vi "Teleop.vi"(10 "Match Info":T1={"Autonomous Elapsed Seconds"=0.0, "TeleOp Elapsed Seconds"=0.0, "Disabled Elapsed Seconds"=0.0, "Visited Autonomous"=FALSE, "Visited TeleOp"=FALSE, "Visited Disabled"=FALSE, "Autonomous Settings"={"Autonomous Style"=enum."Independent", "VI Refnum"=refnum}}, 11 "Call Context":T2) -> ()   [LabVIEW 2013]
doc: "This VI is called for each TeleOp packet received from the DS where the robot is not disabled. It is often used to read from the joysticks and update I/O or to update setpoints for timed control loops. It should complete and return within 20 milliseconds or it may miss DS packets."
uses:
  <vilib>/Rock Robotics/WPI/DriverStation/WPI_DriverStationDerivedRobotMode.ctl
  <vilib>/Rock Robotics/WPI/DriverStation/WPI_DriverStationMatch Info.ctl
  <vilib>/Rock Robotics/WPI/Joystick/WPI_JoystickAxis.ctl
  Robot Global Data.vi
  <vilib>/Rock Robotics/WPI/RobotDrive/WPI_RobotDriveMecanumDrive_Cartesian.vi
  <vilib>/Rock Robotics/WPI/Joystick/WPI_JoystickGetSetRefNum.vi
  <vilib>/Rock Robotics/WPI/RobotDrive/WPI_RobotDriveGetSetRefNum.vi
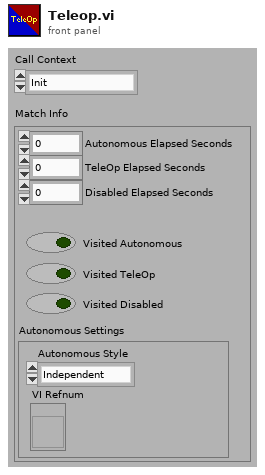
[diagram p1: front panel]
types:
  T1 = typedef "WPI_DriverStationMatch Info.ctl" = cluster{"Autonomous Elapsed Seconds":dbl, "TeleOp Elapsed Seconds":dbl, "Disabled Elapsed Seconds":dbl, "Visited Autonomous":bool, "Visited TeleOp":bool, "Visited Disabled":bool, "Autonomous Settings":cluster{"Autonomous Style":enum16{"Iterative", "Independent"}, "VI Refnum":refnum<vi>}}
  T2 = typedef "WPI_DriverStationDerivedRobotMode.ctl" = enum16{"Init", "Execute", "Stop"}
  T3 = typedef "WPI_JoystickAxis.ctl" = enum16{"Axis 1", "Axis 2", "Axis 3", "Axis 4", "Axis 5", "Axis 6"}
  T4 = typedef "WPI_JoystickDevRef.ctl" = cluster{"Device":T5}
  T5 = typedef "WPI_JoystickDeviceEnum.ctl" = enum16{"USB 1", "USB 2", "USB 3", "USB 4", "Kinect 1", "Kinect 2"}
  T6 = cluster{"axis 1 (x)":dbl, "axis 2 (y)":dbl, "axis 3 (throttle)":dbl, "axis 4":dbl, "axis 5":dbl, "axis 6":dbl}
  T7 = typedef "WPI_AnalogChannelDevRef.ctl" = cluster{"DevStatus":errorcluster, "Analog Module":T8, "Analog Channel":T9}
  T8 = typedef "FPGA_TypedefAnalogModule.ctl" = enum16{"Analog Module 1", "Analog Module 2"}
  T9 = typedef "FPGA_AIChannel.ctl" = enum8{"AI 1", "AI 2", "AI 3", "AI 4", "AI 5", "AI 6", "AI 7", "AI 8", "Invalid"}
  T10 = typedef "WPI_MotorControlDeviceRef.ctl" = cluster{"DeviceStatus":errorcluster, "Type":enum16{"PWM", "CAN"}, "PWM":cluster{"Digital Module":T11, "PWM Channel":T12, "DeadBand":T13}, "CAN":cluster{"Device Number":u8, "Control Mode":T14, "Semaphore":T15, "Max Vout":dbl}, "Invert":bool, "TransformRef":T16, "InvTransformRef":T16}
  T11 = typedef "FPGA_TypedefDigitalModule.ctl" = enum16{"Digital Module 1", "Digital Module 2"}
  T12 = typedef "FPGA_DIOPWMChannel.ctl" = enum8{"PWM 1", "PWM 2", "PWM 3", "PWM 4", "PWM 5", "PWM 6", "PWM 7", "PWM 8", "PWM 9", "PWM 10", "Invalid"}
  T13 = typedef "WPI_PWMDeadband.ctl" = cluster{"Name":string, "maxPositivePwm":i32, "minPositivePwm":i32, "centerPwm":i32, "maxNegativePwm":i32, "minNegativePwm":i32, "angularRange":u16}
  T14 = typedef "WPI_CANJaguar_ControlMode.ctl" = enum8{"Percent VBus", "Current", "Speed", "Position", "Voltage"}
  T15 = typedef "Semaphore RefNum" = refnum<k1>
  T16 = typedef "WPI_PWMTransform_ConPane.ctl" = refnum<vi>
  T17 = typedef "WPI_RobotDriveDevRef.ctl" = cluster{"DevStatus":errorcluster, "Motors[]":T10[], "Square Inputs":bool, "Max Output":dbl, "Isochronous":bool}
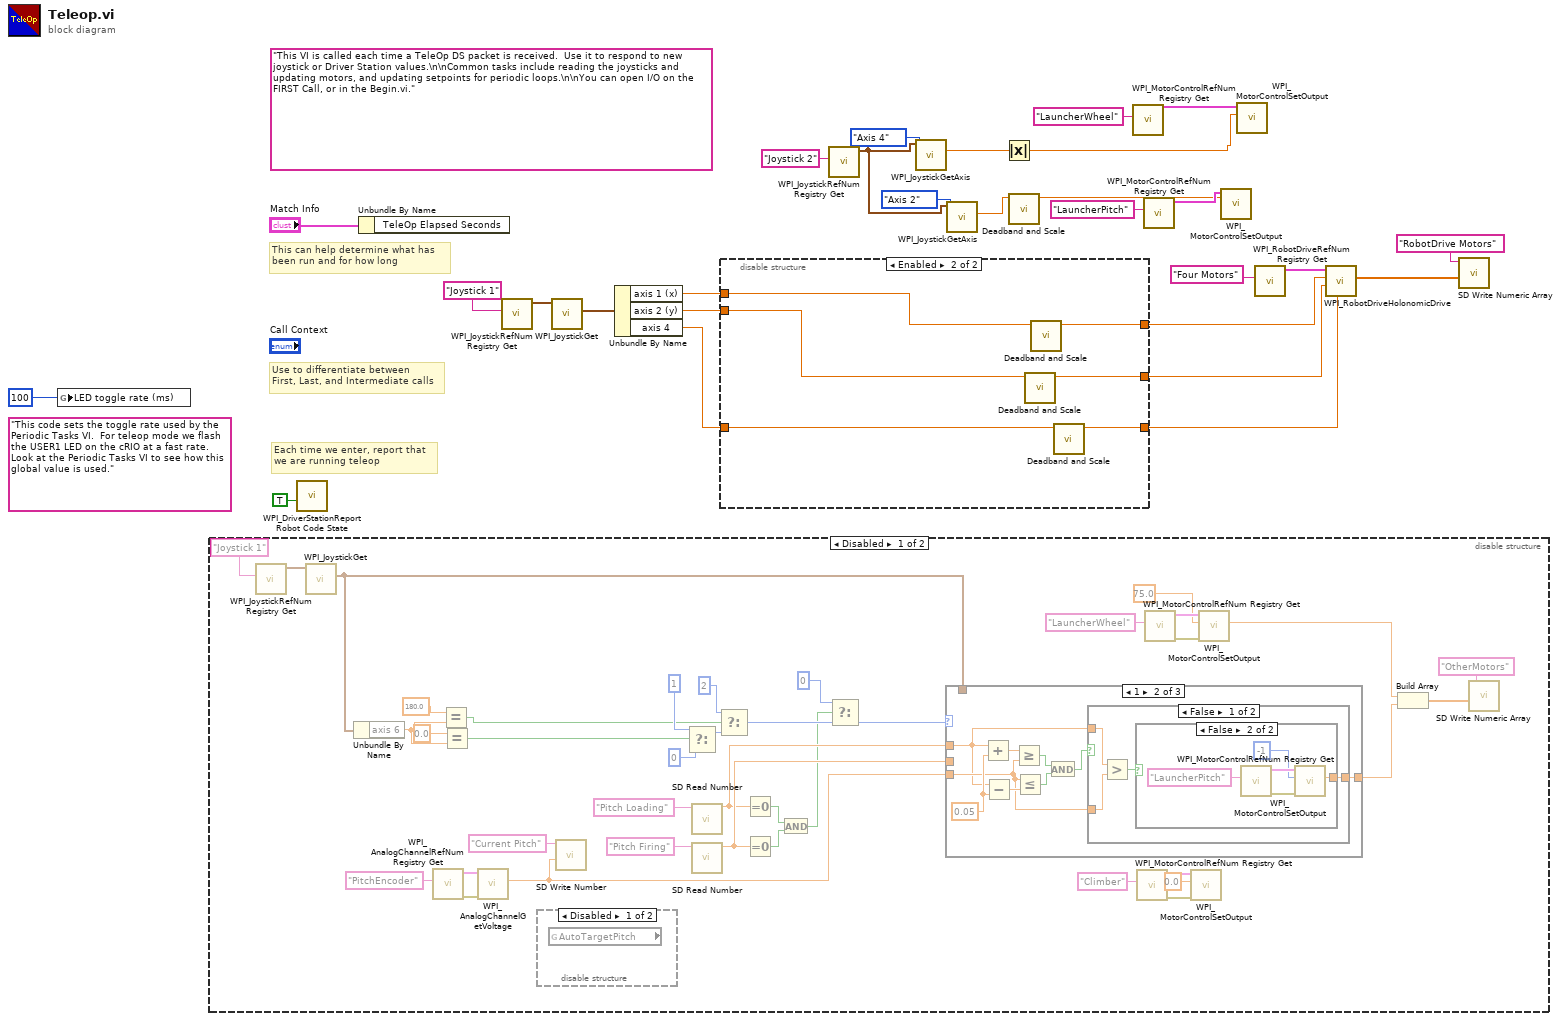
[diagram p0: block diagram]
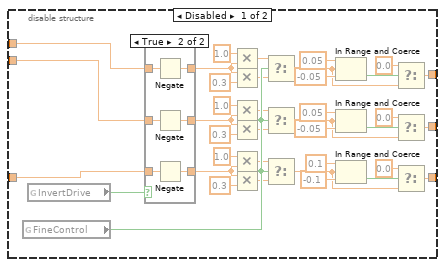
[diagram p2: hidden frame]
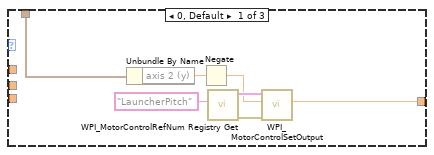
[diagram p4: hidden frame]
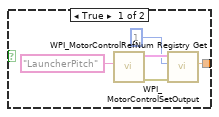
[diagram p5: hidden frame]
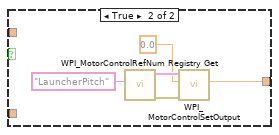
[diagram p6: hidden frame]
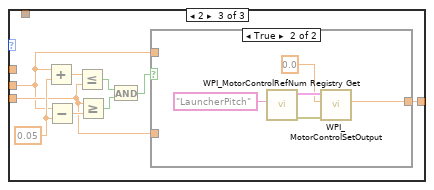
[diagram p7: hidden frame]
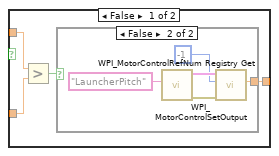
[diagram p8: hidden frame]
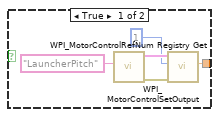
[diagram p9: hidden frame]
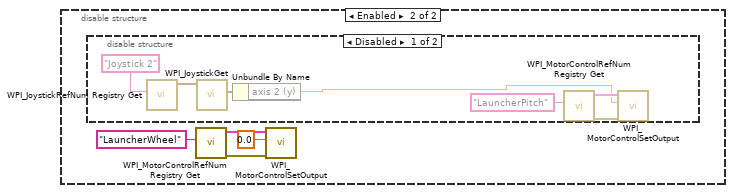
[diagram p11: hidden frame]
diagram:
  (unwired) "This code sets the toggle rate used by the Periodic Tasks VI.  For teleop mode we flash the USER1 LED on the cRIO at a fast rate.  Look at the Periodic Tasks VI to see how this global value is used."
  (unwired) "This VI is called each time a TeleOp DS packet is received.  Use it to respond to new joystick or Driver Station values.\n\nCommon tasks include reading the joysticks and updating motors, and updating setpoints for periodic loops.\n\nYou can open I/O on the FIRST Call, or in the Begin.vi."
  # "Each time we enter, report that\nwe are running teleop"
  # "Use to differentiate between\nFirst, Last, and Intermediate calls"
  # "This can help determine what has\nbeen run and for how long"
  n1 = global write "Robot Global Data.vi" "LED toggle rate (ms)"(u32 100 ("LED ms toggle rate")) -> ()
  n2 = disable-structure shown="Disabled" {
    frame Disabled {
      n3 = call <vilib>:"WPI_JoystickRefNum Registry Get.vi"("refnum name"="Joystick 1") -> ("JoystickDevRef"=w63:T4)  [unwired: 1 in, 9 out]
      n4 = call <vilib>:"WPI_JoystickGet.vi"("JoystickDevRef"=w63) -> ("Axes"=w35:T6)  [unwired: 1 in, 5 out]
      n5 = Unbundle By Name(w35) -> ("axis 6"=w31:dbl)
      n6 = call <vilib>:"WPI_AnalogChannelRefNum Registry Get.vi"("refnum name"="PitchEncoder") -> ("error out"=w58:errorcluster, "AIDeviceRef"=w57:T7)  [unwired: 9 in]
      n7 = Equal?(x=180.0 ("axis 6"), y=w31) -> (x = y?=w32:bool)
      n8 = Equal?(x=0.0, y=w31) -> (x = y?=w30:bool)
      n9 = call <vilib>:"WPI_AnalogChannelGetVoltage.vi"("error in (no error)"=w58, "AIDeviceRef"=w57) -> ("Voltage"=w40:dbl)  [unwired: 7 in, 2 out]
      n10 = disable-structure shown="Disabled" {
        frame Disabled {
          n11 = global read "Robot Global Data.vi" "AutoTargetPitch"() -> ()  [unwired: 1 out]
        }
        frame Enabled {
        }
      }
      n12 = call <vilib>:"SD Write Number.vi"("Numeric"=w40, "Name"="Current Pitch") -> ()  [unwired: 8 in, 2 out]
      n13 = Select(t=1, s=w30, f=0) -> (s? t:f=w53:i32)
      n14 = call <vilib>:"SD Read Number.vi"("Name"="Pitch Loading") -> ("Numeric"=w45:dbl)  [unwired: 8 in, 2 out]
      n15 = call <vilib>:"SD Read Number.vi"("Name"="Pitch Firing") -> ("Numeric"=w46:dbl)  [unwired: 8 in, 2 out]
      n16 = Select(t=2, s=w32, f=w53) -> (s? t:f=w48:i32)
      n17 = Equal To 0?(x=w45) -> (x = 0?=w44:bool)
      n18 = Equal To 0?(x=w46) -> (x = 0?=w43:bool)
      n19 = And(x=w44, y=w43) -> (x .and. y?=w42:bool)
      n20 = Select(t=0, s=w42, f=w48) -> (s? t:f=w47:i32)
      n21 = case shown="1" w47 {
        tunnel: w35 -> [w74 _ _]
        tunnel: [w73 w77 w105] -> w60
        tunnel: w45 -> [_ w75 _]
        tunnel: w46 -> [_ _ w103]
        tunnel: w40 -> [_ w76 w104]
        frame 0, Default {
          n22 = Unbundle By Name(w74) -> ("axis 2 (y)"=w69:dbl)
          n23 = Negate(x=w69) -> (-x=w68:dbl)
          n24 = call <vilib>:"WPI_MotorControlRefNum Registry Get.vi"("refnum name"="LauncherPitch") -> ("error out"=w71:errorcluster, "MotorControlDevRef"=w72:T10)  [unwired: 9 in]
          n25 = call <vilib>:"WPI_MotorControlSetOutput.vi"("error in (no error)"=w71, "Output"=w68, "MotorControlDevRef"=w72) -> ("Motor Output"=w73:dbl)  [unwired: 6 in, 2 out]
        }
        frame 1 {
          w83 = 0.05
          n26 = Add(x=w75, y=w83) -> (x+y=w82:dbl)
          n27 = Subtract(x=w75, y=w83) -> (x-y=w81:dbl)
          n28 = Greater Or Equal?(x=w82, y=w76) -> (x >= y?=w79:bool)
          n29 = Less Or Equal?(x=w76, y=w81) -> (x <= y?=w80:bool)
          n30 = And(x=w79, y=w80) -> (x .and. y?=w78:bool)
          n31 = case shown="False" w78 {
            tunnel: [w84 w99] -> w77
            tunnel: w76 -> [w85 _]
            tunnel: w75 -> [w86 _]
            frame False {
              n32 = Greater?(x=w86, y=w85) -> (0:w87:bool)
              n33 = case shown="False" w87 {
                tunnel: [w89 w94] -> w84
                frame True {
                  n34 = call <vilib>:"WPI_MotorControlRefNum Registry Get.vi"("refnum name"="LauncherPitch") -> ("error out"=w91:errorcluster, "MotorControlDevRef"=w92:T10)  [unwired: 9 in]
                  n35 = call <vilib>:"WPI_MotorControlSetOutput.vi"("error in (no error)"=w91, "Output"=1, "MotorControlDevRef"=w92) -> ("Motor Output"=w89:dbl)  [unwired: 6 in, 2 out]
                }
                frame False {
                  n36 = call <vilib>:"WPI_MotorControlRefNum Registry Get.vi"("refnum name"="LauncherPitch") -> ("error out"=w96:errorcluster, "MotorControlDevRef"=w97:T10)  [unwired: 9 in]
                  n37 = call <vilib>:"WPI_MotorControlSetOutput.vi"("error in (no error)"=w96, "Output"=-1, "MotorControlDevRef"=w97) -> ("Motor Output"=w94:dbl)  [unwired: 6 in, 2 out]
                }
              }
            }
            frame True {
              n38 = call <vilib>:"WPI_MotorControlRefNum Registry Get.vi"("refnum name"="LauncherPitch") -> ("error out"=w101:errorcluster, "MotorControlDevRef"=w102:T10)  [unwired: 9 in]
              n39 = call <vilib>:"WPI_MotorControlSetOutput.vi"("error in (no error)"=w101, "Output"=0.0, "MotorControlDevRef"=w102) -> ("Motor Output"=w99:dbl)  [unwired: 6 in, 2 out]
            }
          }
        }
        frame 2 {
          w111 = 0.05
          n40 = Add(x=w103, y=w111) -> (x+y=w110:dbl)
          n41 = Subtract(x=w103, y=w111) -> (x-y=w109:dbl)
          n42 = Less Or Equal?(x=w110, y=w104) -> (x <= y?=w107:bool)
          n43 = Greater Or Equal?(x=w104, y=w109) -> (x >= y?=w108:bool)
          n44 = And(x=w107, y=w108) -> (x .and. y?=w106:bool)
          n45 = case shown="True" w106 {
            tunnel: [w112 w127] -> w105
            tunnel: w104 -> [w113 _]
            tunnel: w103 -> [w114 _]
            frame False {
              n46 = Greater?(x=w114, y=w113) -> (0:w115:bool)
              n47 = case shown="False" w115 {
                tunnel: [w117 w122] -> w112
                frame True {
                  n48 = call <vilib>:"WPI_MotorControlRefNum Registry Get.vi"("refnum name"="LauncherPitch") -> ("error out"=w119:errorcluster, "MotorControlDevRef"=w120:T10)  [unwired: 9 in]
                  n49 = call <vilib>:"WPI_MotorControlSetOutput.vi"("error in (no error)"=w119, "Output"=1, "MotorControlDevRef"=w120) -> ("Motor Output"=w117:dbl)  [unwired: 6 in, 2 out]
                }
                frame False {
                  n50 = call <vilib>:"WPI_MotorControlRefNum Registry Get.vi"("refnum name"="LauncherPitch") -> ("error out"=w124:errorcluster, "MotorControlDevRef"=w125:T10)  [unwired: 9 in]
                  n51 = call <vilib>:"WPI_MotorControlSetOutput.vi"("error in (no error)"=w124, "Output"=-1, "MotorControlDevRef"=w125) -> ("Motor Output"=w122:dbl)  [unwired: 6 in, 2 out]
                }
              }
            }
            frame True {
              n52 = call <vilib>:"WPI_MotorControlRefNum Registry Get.vi"("refnum name"="LauncherPitch") -> ("error out"=w129:errorcluster, "MotorControlDevRef"=w130:T10)  [unwired: 9 in]
              n53 = call <vilib>:"WPI_MotorControlSetOutput.vi"("error in (no error)"=w129, "Output"=0.0, "MotorControlDevRef"=w130) -> ("Motor Output"=w127:dbl)  [unwired: 6 in, 2 out]
            }
          }
        }
      }
      n54 = call <vilib>:"WPI_MotorControlRefNum Registry Get.vi"("refnum name"="Climber") -> ("error out"=w38:errorcluster, "MotorControlDevRef"=w39:T10)  [unwired: 9 in]
      n55 = call <vilib>:"WPI_MotorControlRefNum Registry Get.vi"("refnum name"="LauncherWheel") -> ("error out"=w66:errorcluster, "MotorControlDevRef"=w67:T10)  [unwired: 9 in]
      n56 = call <vilib>:"WPI_MotorControlSetOutput.vi"("error in (no error)"=w38, "Output"=0.0, "MotorControlDevRef"=w39) -> ()  [unwired: 6 in, 3 out]
      n57 = call <vilib>:"WPI_MotorControlSetOutput.vi"("error in (no error)"=w66, "Output"=75.0, "MotorControlDevRef"=w67) -> ("Motor Output"=w59:dbl)  [unwired: 6 in, 2 out]
      n58 = Build Array(w59, w60) -> (w61:dbl[])
      n59 = call <vilib>:"SD Write Numeric Array.vi"("Numeric Array"=w61, "Name"="OtherMotors") -> ()  [unwired: 8 in, 2 out]
    }
    frame Enabled {
      n60 = disable-structure shown="Disabled" {
        frame Disabled {
          n61 = call <vilib>:"WPI_JoystickRefNum Registry Get.vi"("refnum name"="Joystick 2") -> ("JoystickDevRef"=w140:T4)  [unwired: 1 in, 9 out]
          n62 = call <vilib>:"WPI_JoystickGet.vi"("JoystickDevRef"=w140) -> ("Axes"=w139:T6)  [unwired: 1 in, 5 out]
          n63 = Unbundle By Name(w139) -> ("axis 2 (y)"=w135:dbl)
          n64 = call <vilib>:"WPI_MotorControlRefNum Registry Get.vi"("refnum name"="LauncherPitch") -> ("error out"=w137:errorcluster, "MotorControlDevRef"=w138:T10)  [unwired: 9 in]
          n65 = call <vilib>:"WPI_MotorControlSetOutput.vi"("error in (no error)"=w137, "Output"=w135, "MotorControlDevRef"=w138) -> ()  [unwired: 6 in, 3 out]
        }
        frame Enabled {
        }
      }
      n66 = call <vilib>:"WPI_MotorControlRefNum Registry Get.vi"("refnum name"="LauncherWheel") -> ("error out"=w133:errorcluster, "MotorControlDevRef"=w134:T10)  [unwired: 9 in]
      n67 = call <vilib>:"WPI_MotorControlSetOutput.vi"("error in (no error)"=w133, "Output"=0.0, "MotorControlDevRef"=w134) -> ()  [unwired: 6 in, 3 out]
    }
  }
  n68 = call <vilib>:"WPI_DriverStationReport Robot Code State.vi"("TeleOp"=TRUE ("Autonomous")) -> ()  [unwired: 10 in, 1 out]
  n69 = Unbundle By Name("Match Info") -> ()  [unwired: 1 out]
  n70 = call <vilib>:"WPI_JoystickRefNum Registry Get.vi"("refnum name"="Joystick 1") -> ("JoystickDevRef"=w24:T4)  [unwired: 1 in, 9 out]
  n71 = call <vilib>:"WPI_JoystickGet.vi"("JoystickDevRef"=w24) -> ("Axes"=w23:T6)  [unwired: 1 in, 5 out]
  n72 = Unbundle By Name(w23) -> ("axis 1 (x)"=w15:dbl, "axis 2 (y)"=w14:dbl, "axis 4"=w13:dbl)
  n73 = disable-structure shown="Enabled" {
    disable-tunnel: [w150 w189] -> w18
    disable-tunnel: [w149 w190] -> w17
    disable-tunnel: [w148 w191] -> w16
    disable-tunnel: w15 -> [w144 w194]
    disable-tunnel: w14 -> [w143 w193]
    disable-tunnel: w13 -> [w142 w192]
    frame Disabled {
      n74 = global read "Robot Global Data.vi" "FineControl"() -> (w179:bool)
      n75 = global read "Robot Global Data.vi" "InvertDrive"() -> (w178:bool)
      n76 = case shown="True" w178 {
        tunnel: [w181 w188] -> w147
        tunnel: [w180 w187] -> w146
        tunnel: [w182 w186] -> w145
        tunnel: w144 -> [w182 w185]
        tunnel: w143 -> [w181 w184]
        tunnel: w142 -> [w180 w183]
        frame False {
        }
        frame True {
          n77 = Negate(x=w185) -> (-x=w186:dbl)
          n78 = Negate(x=w184) -> (-x=w188:dbl)
          n79 = Negate(x=w183) -> (-x=w187:dbl)
        }
      }
      n80 = Multiply(x=1.0, y=w145) -> (x*y=w165:dbl)
      n81 = Multiply(x=w145, y=0.3) -> (x*y=w164:dbl)
      n82 = Multiply(x=1.0, y=w147) -> (x*y=w174:dbl)
      n83 = Multiply(x=w147, y=0.3) -> (x*y=w173:dbl)
      n84 = Multiply(x=1.0, y=w146) -> (x*y=w157:dbl)
      n85 = Multiply(x=w146, y=0.3) -> (x*y=w156:dbl)
      n86 = Select(t=w165, s=w179, f=w164) -> (s? t:f=w161:dbl)
      n87 = Select(t=w174, s=w179, f=w173) -> (s? t:f=w170:dbl)
      n88 = Select(t=w157, s=w179, f=w156) -> (s? t:f=w153:dbl)
      n89 = In Range and Coerce(upper limit=0.05, x=w161, lower limit=-0.05) -> (In Range?=w162:bool)  [unwired: 1 out]
      n90 = In Range and Coerce(upper limit=0.05, x=w170, lower limit=-0.05) -> (In Range?=w169:bool)  [unwired: 1 out]
      n91 = In Range and Coerce(upper limit=0.1, x=w153, lower limit=-0.1) -> (In Range?=w152:bool)  [unwired: 1 out]
      n92 = Select(t=0.0, s=w162, f=w161) -> (s? t:f=w150:dbl)
      n93 = Select(t=0.0, s=w169, f=w170) -> (s? t:f=w149:dbl)
      n94 = Select(t=0.0, s=w152, f=w153) -> (s? t:f=w148:dbl)
    }
    frame Enabled {
      n95 = call "Deadband and Scale.vi"("Input"=w193) -> ("Output"=w190:dbl)  [unwired: 10 in]
      n96 = call "Deadband and Scale.vi"("Input"=w194) -> ("Output"=w189:dbl)  [unwired: 10 in]
      n97 = call "Deadband and Scale.vi"("Input"=w192) -> ("Output"=w191:dbl)  [unwired: 10 in]
    }
  }
  n98 = call <vilib>:"WPI_JoystickRefNum Registry Get.vi"("refnum name"="Joystick 2") -> ("JoystickDevRef"=w7:T4)  [unwired: 9 in, 1 out]
  n99 = call <vilib>:"WPI_JoystickGetAxis.vi"("Axis"=WPI_JoystickAxis."Axis 4", "JoystickDevRef"=w7) -> ("Value"=w6:dbl)  [unwired: 8 in, 1 out]
  n100 = call <vilib>:"WPI_JoystickGetAxis.vi"("Axis"=WPI_JoystickAxis."Axis 2", "JoystickDevRef"=w7) -> ("Value"=w1:dbl)  [unwired: 8 in, 1 out]
  n101 = Absolute Value(x=w6) -> (abs(x)=w5:dbl)
  n102 = call "Deadband and Scale.vi"("Input"=w1) -> ("Output"=w2:dbl)  [unwired: 10 in]
  n103 = call <vilib>:"WPI_MotorControlRefNum Registry Get.vi"("refnum name"="LauncherWheel") -> ("MotorControlDevRef"=w12:T10)  [unwired: 9 in, 1 out]
  n104 = call <vilib>:"WPI_MotorControlRefNum Registry Get.vi"("refnum name"="LauncherPitch") -> ("MotorControlDevRef"=w3:T10)  [unwired: 9 in, 1 out]
  n105 = call <vilib>:"WPI_MotorControlSetOutput.vi"("Output"=w2, "MotorControlDevRef"=w3) -> ()  [unwired: 7 in, 3 out]
  n106 = call <vilib>:"WPI_MotorControlSetOutput.vi"("Output"=w5, "MotorControlDevRef"=w12) -> ()  [unwired: 7 in, 3 out]
  n107 = call <vilib>:"WPI_RobotDriveRefNum Registry Get.vi"("refnum name"="Four Motors") -> ("RobotDriveDevRef"=w19:T17)  [unwired: 1 in, 9 out]
  n108 = call-poly <vilib>:"WPI_RobotDriveHolonomicDrive.vi"("Rotation"=w16, "Y"=w17, "X"=w18, "RobotDriveDevRef"=w19) -> ("Motor Values"=w22:dbl[])  [unwired: 5 in, 2 out]
  n109 = call <vilib>:"SD Write Numeric Array.vi"("Numeric Array"=w22, "Name"="RobotDrive Motors") -> ()  [unwired: 8 in, 2 out]
